vi "Uint32 Create.vi"(8 "error in (no error)":errorcluster, 11 "U32 in":u32) -> (0 "error out":errorcluster, 3 "Uint32 DVR out":refnum<data-value>)   [LabVIEW 2012, in "MDSplus.lvlib"]
uses:
  <vilib>/MDSplus/Library/MDSplus.lvlib
  <vilib>/MDSplus/Classes/Data_Class/Scalar_Class/Uint32_Class/Uint32.lvclass
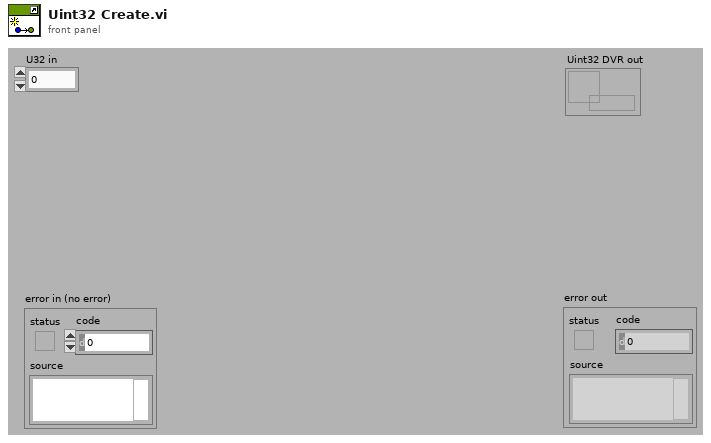
[diagram p1: front panel]
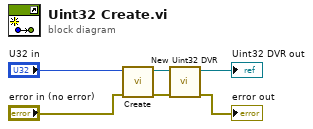
[diagram p0: block diagram]
diagram:
  n1 = call <vilib>:"Create.vi"("error in (no error)"="error in (no error)", "U32 in"="U32 in") -> ("error out"=w3:errorcluster, "Uint32 out"=w4:refnum<class "Uint32.lvclass">)  [unwired: 8 in]
  n2 = call <vilib>:"New Uint32 DVR.vi"("error in (no error)"=w3, "Uint32 in"=w4) -> ("error out"=→"error out":errorcluster, "Uint32 DVR out"=→"Uint32 DVR out":refnum<data-value>)  [unwired: 8 in]
